vi "get_LSID.vi"(8 "error in (no error)":errorcluster, 10 "namespace":string, 11 "GenericPlugin in":refnum<class "GenericComponent.lvclass">) -> (0 "error out":errorcluster, 1 "LSID (cluster)":T1, 2 "LSID (string)":string, 3 "GenericPlugin out":refnum<class "GenericComponent.lvclass">)   [LabVIEW 2010, in "GenericComponent.lvclass"]
uses:
  GenericComponent.lvclass
  clusters/LSID_cluster.ctl
  GenericComponent.lvclass/GenericComponent.ctl
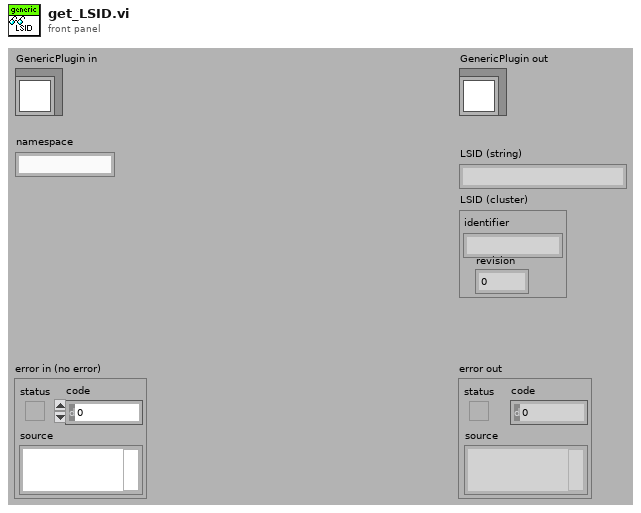
[diagram p1: front panel]
types:
  T1 = typedef "LSID_cluster.ctl" = cluster{"identifier":string, "revision":i32}
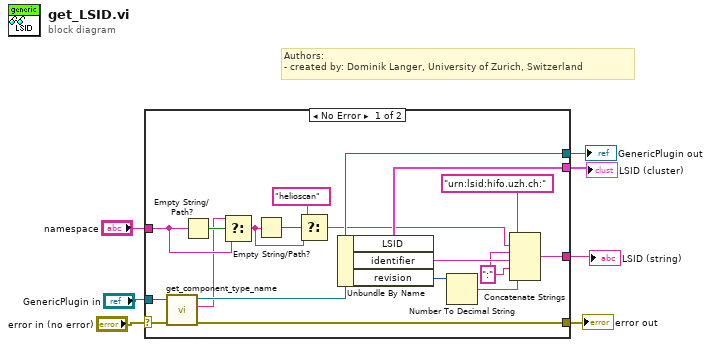
[diagram p0: block diagram]
diagram:
  # "Authors: \n- created by: Dominik Langer, University of Zurich, Switzerland"
  n1 = case shown="No Error" "error in (no error)" {
    selector: "error in (no error)" -> [w16 w27]
    tunnel: [w15 w27] -> w6
    tunnel: [w13 w26] -> w4
    tunnel: "GenericPlugin in" -> [w14 w26]
    tunnel: [w24 _] -> w3
    tunnel: [w21 _] -> w2
    tunnel: "namespace" -> [w18 _]
    frame No Error {
      w17 = ":"
      n2 = call-dynamic "get_component_type_name.vi"("error in (no error)"=w16, "GenericPlugin in"=w14) -> ("error out"=w15:errorcluster, "component type"=w12:string, "GenericPlugin out"=w13:refnum<class "GenericComponent.lvclass">)  [unwired: 7 in]
      n3 = Empty String/Path?(string/path=w18) -> (empty?=w19:bool)
      n4 = Select(t=w12, s=w19, f=w18) -> (s? t:f=w10:string)
      n5 = Empty String/Path?(string/path=w10) -> (empty?=w11:bool)
      n6 = Select(t="helioscan", s=w11, f=w10) -> (s? t:f=w8:string)
      n7 = Unbundle By Name(w13) -> ("LSID"=w21:T1, "identifier"=w22:string, "revision"=w23:i32)
      n8 = Number To Decimal String(number=w23) -> (decimal integer string=w25:string)  [unwired: 1 in]
      n9 = Concatenate Strings("urn:lsid:hifo.uzh.ch:" ("string"), w8, w17, w22, w17, w25) -> (w24:string)
    }
    frame Error {
    }
  }
  "error out" <- w6
  "GenericPlugin out" <- w4
  "LSID (string)" <- w3
  "LSID (cluster)" <- w2
